vi "Finish Comment.vi"(7 "QRD":T1, 8 "error in":errorcluster) -> (0 "error out":errorcluster, 5 "QRD Out":T1)   [LabVIEW 2025]
uses:
  Builds/Queue Wrappers.lvlibp
  Builds/Queue Wrappers.lvlibp/Q Packet.ctl
  Controls/Queues-Refs-Data.ctl
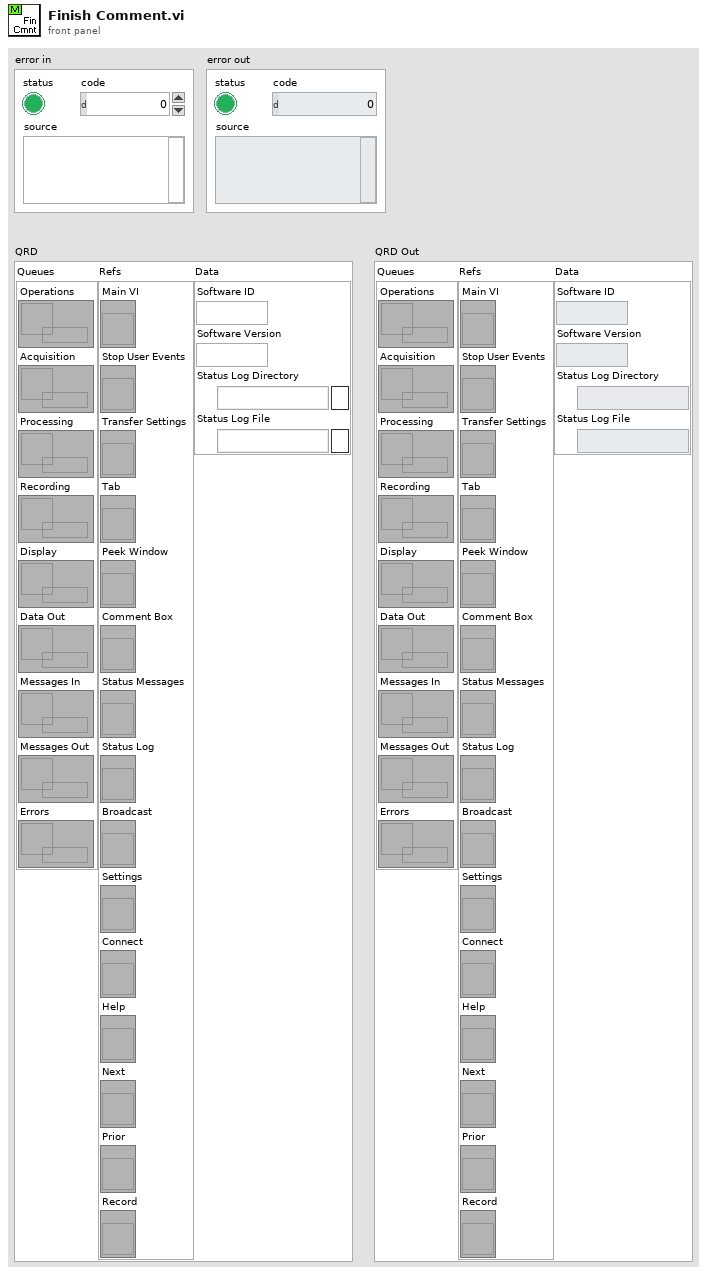
[diagram p1: front panel]
types:
  T1 = typedef "Queues-Refs-Data.ctl" = cluster{"Queues":cluster{"Operations":refnum<queue>, "Acquisition":refnum<queue>, "Processing":refnum<queue>, "Recording":refnum<queue>, "Display":refnum<queue>, "Data Out":refnum<queue>, "Messages In":refnum<queue>, "Messages Out":refnum<queue>, "Errors":refnum<queue>}, "Refs":cluster{"Main VI":refnum<vi>, "Stop User Events":refnum<vi>, "Transfer Settings":refnum<vi>, "Tab":refnum<vi>, "Peek Window":refnum<vi>, "Comment Box":refnum<vi>, "Status Messages":refnum<vi>, "Status Log":refnum<vi>, "Broadcast":refnum<vi>, "Settings":refnum<vi>, "Connect":refnum<vi>, "Help":refnum<vi>, "Next":refnum<vi>, "Prior":refnum<vi>, "Record":refnum<vi>}, "Data":cluster{"Software ID":string, "Software Version":string, "Status Log Directory":path, "Status Log File":path}}
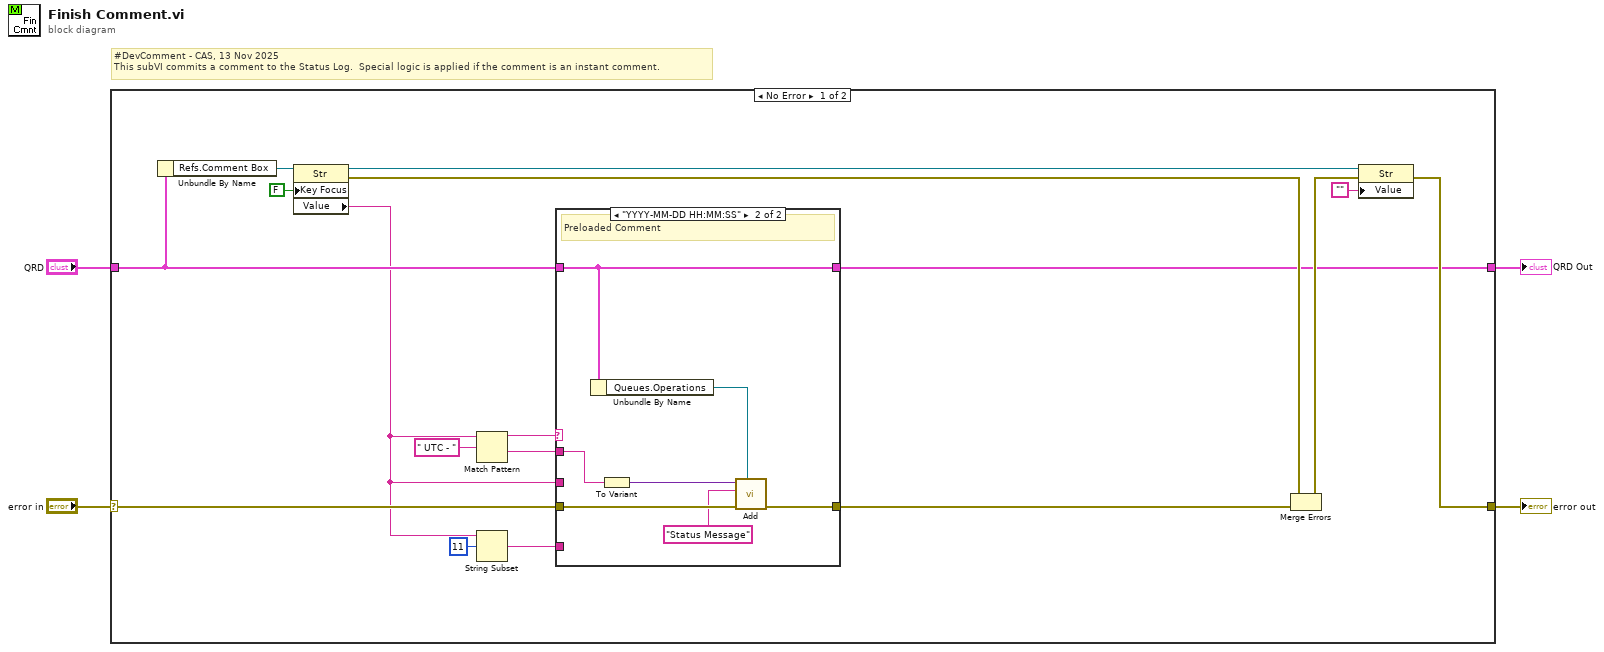
[diagram p0: block diagram]
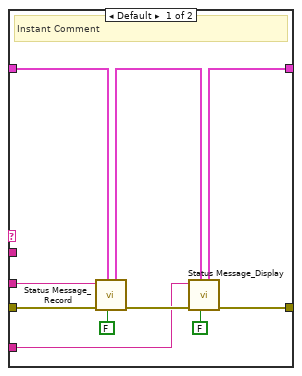
[diagram p2: hidden frame]
diagram:
  # "#DevComment - CAS, 13 Nov 2025\nThis subVI commits a comment to the Status Log.  Special logic is applied if the comment is an instant comment."
  n1 = case shown="No Error" "error in" {
    selector: "error in" -> [w15 w40]
    tunnel: "QRD" -> [w9 w39]
    tunnel: [w11 w40] -> w2
    tunnel: [w10 w39] -> w1
    frame No Error {
      n2 = Unbundle By Name(w9) -> ("Refs.Comment Box"=w21:refnum<vi>)
      n3 = property class="Str"(reference=w21, "Key Focus"=FALSE) -> (reference out=w20:refnum<vi>, error out=w13:errorcluster, "Value"=w7:string)  [unwired: 1 in]
      n4 = Match Pattern(string=w7, regular expression=" UTC - ") -> (before substring=w17:string, after substring=w16:string)  [unwired: 1 in, 2 out]
      n5 = String Subset(string=w7, offset (0)=11) -> (substring=w6:string)  [unwired: 1 in]
      n6 = case shown="\"YYYY-MM-DD HH:MM:SS\"" w17 {
        tunnel: w16 -> [_ w34]
        tunnel: w15 -> [w30 w38]
        tunnel: w9 -> [w28 w35]
        tunnel: [w29 w36] -> w14
        tunnel: [w26 w35] -> w10
        tunnel: w7 -> [w24 _]
        tunnel: w6 -> [w22 _]
        frame Default {
          # "Instant Comment"
          n7 = call "Status Message_Record.vi"("Add Timestamp (?)"=FALSE, "QRD"=w28, "error in"=w30, "Status Message"=w24) -> ("error out"=w31:errorcluster, "QRD Out"=w27:T1)  [unwired: 5 in, 1 out]
          n8 = call "Status Message_Display.vi"("Add Timestamp (?)"=FALSE, "QRD"=w27, "error in"=w31, "Status Message"=w22) -> ("error out"=w29:errorcluster, "QRD Out"=w26:T1)  [unwired: 6 in]
        }
        frame "YYYY-MM-DD HH:MM:SS" {
          # "Preloaded Comment"
          n9 = Unbundle By Name(w35) -> ("Queues.Operations"=w37:refnum<queue>)
          n10 = To Variant(anything=w34) -> (Variant=w32:variant)
          n11 = call "Add.vi"("Q Ref In"=w37, "error in"=w38, "Message ID"="Status Message" ("Packet ID"), "Payload"=w32) -> ("error out"=w36:errorcluster)  [unwired: 4 in, 3 out]
        }
      }
      n12 = Merge Errors(w13, w14) -> (w12:errorcluster)
      n13 = property class="Str"(reference=w20, error in=w12, "Value"="") -> (error out=w11:errorcluster)  [unwired: 1 out]
    }
    frame Error {
    }
  }
  "error out" <- w2
  "QRD Out" <- w1
